vi "System Options.vi"(7 "Message Text (Empty)":string, 8 "error in (no error)":errorcluster, 9 "Beeper (1:On)":u16(ring)=1 items=["Off", "On", "Once"], 10 "Display (3:On)":enum16{"Clear", "Message", "Off", "On"}(ring)=enum."On", 11 "VISA resource name":refnum<visa-resource-name>) -> (0 "error out":errorcluster, 3 "VISA resource name out":refnum<visa-resource-name>)   [LabVIEW 2013, in "3458A Virtual Digitizer.lvlib" / "3458A Basic Driver.lvlib"]
doc: "Sets Beeper and Display options of the DMM"
uses:
  3458A Basic Driver.lvlib
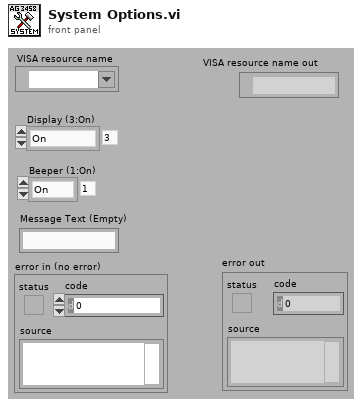
[diagram p1: front panel]
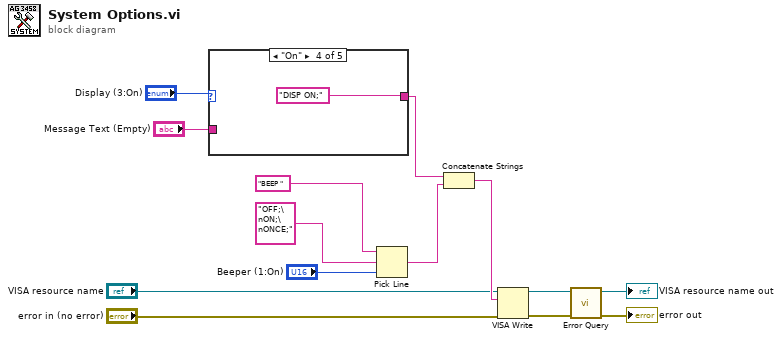
[diagram p0: block diagram]
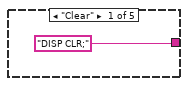
[diagram p2: hidden frame]
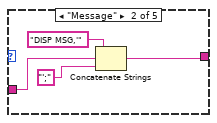
[diagram p3: hidden frame]
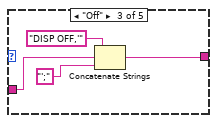
[diagram p4: hidden frame]
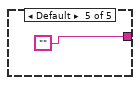
[diagram p5: hidden frame]
diagram:
  n1 = case shown="\"On\"" "Display (3:On)" {
    tunnel: "Message Text (Empty)" -> [_ w17 w20 _ _]
    tunnel: ["DISP CLR;" w16 w21 "DISP ON;" "" ("Empty String Constant")] -> w10
    frame "Clear" {
    }
    frame "Message" {
      n2 = Concatenate Strings("DISP MSG,'", w17, "';") -> (w16:string)
    }
    frame "Off" {
      n3 = Concatenate Strings("DISP OFF,'", w20, "';") -> (w21:string)
    }
    frame "On" {
    }
    frame Default {
    }
  }
  n4 = Pick Line(string ("")="BEEP ", multi-line string="OFF;\nON;\nONCE;", line index="Beeper (1:On)") -> (output string=w9:string)
  n5 = Concatenate Strings(w10, w9) -> (w8:string)
  n6 = VISA Write(VISA resource name="VISA resource name", write buffer=w8, error in (no error)="error in (no error)") -> (VISA resource name out=w14:refnum<visa-resource-name>, error out=w13:errorcluster)  [unwired: 1 out]
  n7 = call "Error Query.vi"("error in (no error)"=w13, "VISA resource name"=w14) -> ("error out"=→"error out":errorcluster, "VISA resource name out"=→"VISA resource name out":refnum<visa-resource-name>)  [unwired: 6 in, 2 out]
